vi "DisplayTemp_channel_writer.vi"() -> ()   [LabVIEW 2017]
uses:
  <extravilib>/ChannelInstances/Stream-c(a[.](str),bool)/Read With Abort.vi
  <extravilib>/ChannelInstances/Stream-c(a[.](str),bool)/Write With Abort.vi
  <extravilib>/ChannelInstances/Stream-c(a[.](str),bool)/EndpointRead.vi
  <extravilib>/ChannelInstances/Stream-c(a[.](str),bool)/Endpoint.vi
  <vilib>/Utility/file.llb/Write Delimited Spreadsheet (string).vi
  <extravilib>/ChannelInstances/Stream-c(a[.](str),bool)/Instantiate.vi
  <extravilib>/ChannelInstances/Stream-c(a[.](str),bool)/)Channel.vi
  <resource>/ChannelSupport/_ChannelSupport/WaitIfNeeded.vi
  <extravilib>/ChannelInstances/Stream-c(a[.](str),bool).lvlib
panel:
  out "date/time string":string
  in  "file path (dialog if empty)":path
  out "Alarm":bool
  in  "Temp treshold":dbl
  out "Celsius Chart":cluster{"Temp treshold":dbl, "C temp":dbl}(graph)
  out "Celsius":dbl(slide) scale=0.0..100.0
  in  "C/F switch":bool
  out "Real\nactual time (ms)":u32
  out "Real \ncycle time (ms)":u32
  out "Computed\nactual time (ms)":u32
  in  "Max time (s)":dbl=10.0
  in  "stop":bool
  out "Farhenheit Chart":dbl(graph)
  out "Farhenheit":dbl(slide) scale=0.0..100.0
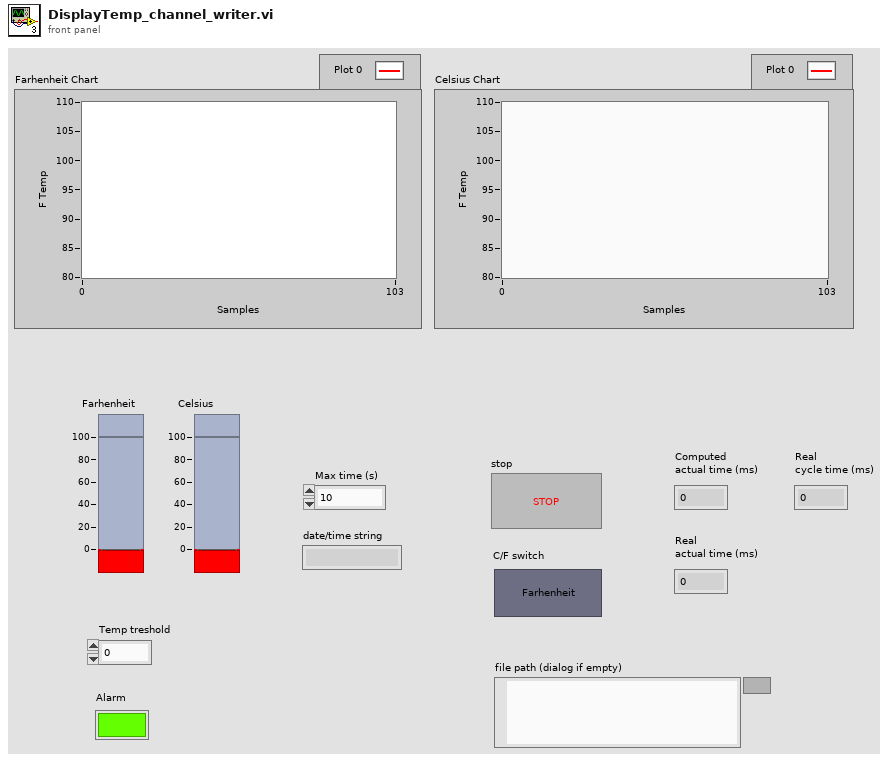
[diagram p1: front panel]
types:
  T1 = typedef "Stream-c(a[.](str),bool).lvlib/)Channel.ctl" = refnum<queue>
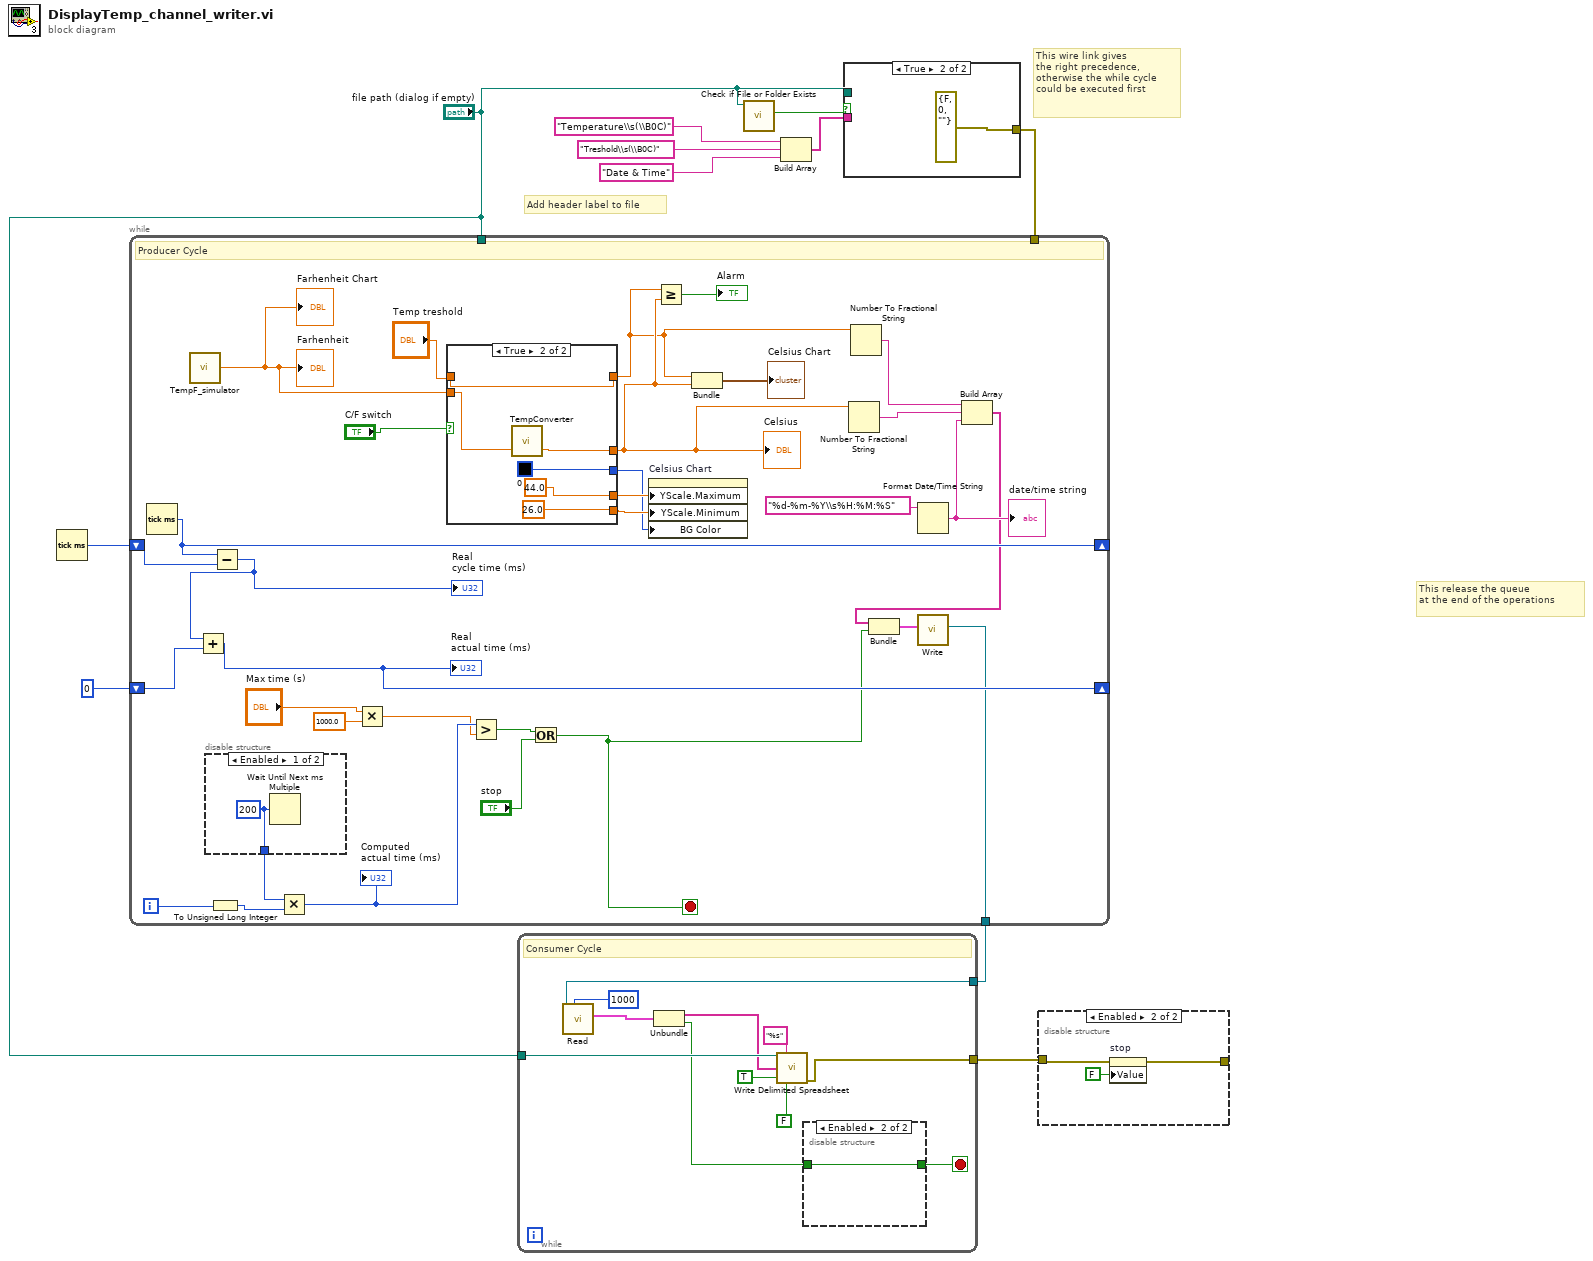
[diagram p0: block diagram]
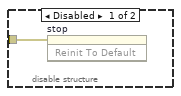
[diagram p2: hidden frame]
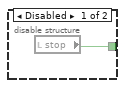
[diagram p3: hidden frame]
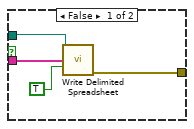
[diagram p4: hidden frame]
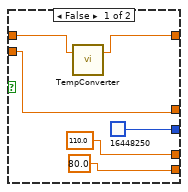
[diagram p5: hidden frame]
diagram:
  # "This release the queue\nat the end of the operations"
  # "This wire link gives\nthe right precedence,\notherwise the while cycle\ncould be executed first"
  # "Add header label to file"
  n1 = Tick Count (ms)() -> (millisecond timer value=w11:u32)
  n2 = call <vilib>:"Check if File or Folder Exists.vi"("path"="file path (dialog if empty)") -> ("file or folder exists?"=w4:bool)  [unwired: 8 in, 2 out]
  n3 = Build Array("Temperature\\s(\\B0C)", "Treshold\\s(\\B0C)" ("element"), "Date & Time" ("element")) -> (w8:string[])
  n4 = case shown="True" w4 {
    tunnel: w8 -> [w15 _]
    tunnel: "file path (dialog if empty)" -> [w14 _]
    tunnel: [w12 errorcluster {"status"=FALSE, "code"=0, "source"=""} ("error out")] -> w5
    frame False {
      n5 = call-poly <vilib>:"Write Delimited Spreadsheet.vi"("file path (dialog if empty)"=w14, "1D data"=w15, "append to file? (new file:F)"=TRUE) -> ("error out"=w12:errorcluster)  [unwired: 11 in, 1 out]
    }
    frame True {
    }
  }
  n6 = while {
    shift-right: [w38] -> _
    shift-left: w11 -> [w39]
    shift-right: [w35] -> _
    shift-left: 0 -> [w37]
    tunnel: "file path (dialog if empty)" -> [_]
    tunnel: w5 -> [_]
    tunnel: [w17] -> w1
    i -> [w42]
    stop <- w19 stop-if-true
    # "Producer Cycle"
    n7 = Tick Count (ms)() -> (millisecond timer value=w38:u32)
    n8 = call "TempF_simulator.vi"() -> ("Farhenheit"=w33:dbl)  [unwired: 1 in]
    "Farhenheit" <- w33
    "Farhenheit Chart" <- w33
    n9 = disable-structure shown="Enabled" {
      disable-tunnel: [w61 _] -> w45
      frame Enabled {
        w61 = u32 200 ("millisecond multiple")
        n10 = Wait Until Next ms Multiple(millisecond multiple=w61) -> ()  [unwired: 1 out]
      }
      frame Disabled {
      }
    }
    n11 = To Unsigned Long Integer(number=w42) -> (unsigned 32bit integer=w41:u32)
    n12 = Subtract(x=w38, y=w39) -> (x-y=w36:u32)
    "Real \ncycle time (ms)" <- w36
    n13 = Add(x=w36, y=w37) -> (x+y=w35:u32)
    "Real\nactual time (ms)" <- w35
    n14 = Multiply(x=w45, y=w41) -> (x*y=w43:u32)
    "Computed\nactual time (ms)" <- w43
    n15 = Multiply(x="Max time (s)", y=1000.0) -> (x*y=w40:dbl)
    n16 = case shown="True" "C/F switch" {
      tunnel: w33 -> [w54 w60]
      tunnel: [w54 w59] -> w24
      tunnel: "Temp treshold" -> [w53 w58]
      tunnel: [w52 w58] -> w23
      tunnel: [110.0 44.0] -> w29
      tunnel: [80.0 26.0] -> w28
      tunnel: [u32 16448250 ("Color Box") u32 0 ("Color Box")] -> w27
      frame False {
        n17 = call "TempConverter.vi"("C temp"=w53) -> ("F temp"=w52:dbl)  [unwired: 1 in, 1 out]
      }
      frame True {
        n18 = call "TempConverter.vi"("F temp"=w60) -> ("C temp"=w59:dbl)  [unwired: 1 in, 1 out]
      }
    }
    "Celsius" <- w24
    n19 = Greater?(x=w43, y=w40) -> (0:w46:bool)
    n20 = Or(x=w46, y="stop") -> (x .or. y?=w19:bool)
    n21 = property on="Celsius Chart" class="WFChart (strict)"("YScale.Maximum"=w29, "YScale.Minimum"=w28, "BG Color"=w27) -> ()  [unwired: 2 in, 2 out]
    n22 = Greater Or Equal?(x=w23, y=w24) -> (x >= y?=→"Alarm":bool)
    n23 = Bundle("Temp treshold"=w23, "C temp"=w24) -> (→"Celsius Chart":cluster{"Temp treshold":dbl, "C temp":dbl})  [unwired: 1 in]
    n24 = Number To Fractional String(number=w24) -> (F-format string=w22:string)  [unwired: 3 in]
    n25 = Number To Fractional String(number=w23) -> (F-format string=w21:string)  [unwired: 3 in]
    n26 = Format Date/Time String(time format string (%c)="%d-%m-%Y\\s%H:%M:%S") -> (date/time string=w25:string)  [unwired: 2 in]
    "date/time string" <- w25
    n27 = Build Array(w21, w22, w25) -> (w20:string[])
    n28 = Bundle(w20, w19) -> (w18:cluster{string[], bool})  [unwired: 1 in]
    n29 = call <extravilib>:"Write.vi"("element"=w18) -> ("channel"=w17:T1)  [unwired: 8 in, 2 out]
  }
  n30 = while {
    tunnel: "file path (dialog if empty)" -> [w69]
    tunnel: [w68] -> w2
    tunnel: w1 -> [w64]
    stop <- w67 stop-if-true
    # "Consumer Cycle"
    n31 = call <extravilib>:"Read.vi"("timeout in ms (-1)"=1000, "channel"=w64) -> ("element"=w63:cluster{string[], bool})  [unwired: 5 in, 4 out]
    n32 = Unbundle(w63) -> (w65:string[], w66:bool)
    n33 = call-poly <vilib>:"Write Delimited Spreadsheet.vi"("file path (dialog if empty)"=w69, "format (%s)"="%s" ("format (%.3f)"), "1D data"=w65, "append to file? (new file:F)"=TRUE, "transpose? (no:F)"=FALSE) -> ("error out"=w68:errorcluster)  [unwired: 9 in, 1 out]
    n34 = disable-structure shown="Enabled" {
      disable-tunnel: [w73 w74] -> w67
      disable-tunnel: w66 -> [_ w74]
      frame Disabled {
        n35 = local read "stop"() -> (w73:bool)
      }
      frame Enabled {
      }
    }
  }
  n36 = disable-structure shown="Enabled" {
    disable-tunnel: w2 -> [w75 w78]
    disable-tunnel: [_ w76] -> _
    frame Disabled {
      n37 = invoke on="stop" class="Bool (strict)" method="Reinit To Default"(error in=w75) -> ()  [unwired: 2 in, 3 out]
    }
    frame Enabled {
      n38 = property on="stop" class="Bool (strict)"(error in=w78, "Value"=FALSE ("stop")) -> (error out=w76:errorcluster)  [unwired: 1 in, 1 out]
    }
  }
